vi "FTW-Regex.vi"(0 "Regular Expression":string, 5 "Input String":string, 9 "Starting Offset":i32, 11 "error in":errorcluster) -> (4 "Match":string, 6 "Submatches":string[](array[string]), 8 "Match Found?":bool, 10 "Offset after Match":i32, 15 "error out":errorcluster)   [LabVIEW 2015]
uses:
  error/FTW-ERR-ThrowGenericError.vi
  error/FTW-ERR-ThrowError.vi
  error/FTW-ERR-CallChain.vi
  error/FTW-ERR-NoErrorConstant.vi
  string/FTW-STR-ReplaceWhitespace.vi
  string/FTW-STR-Array-Delimit.vi
  error/FTW-ERR-Clear.vi
  FTW-Regex-ReplaceAll.vi
  lib/FTW-KernelFilepath.vi
panel:
  # "Inputs"
  # "Debug"
  # "Outputs"
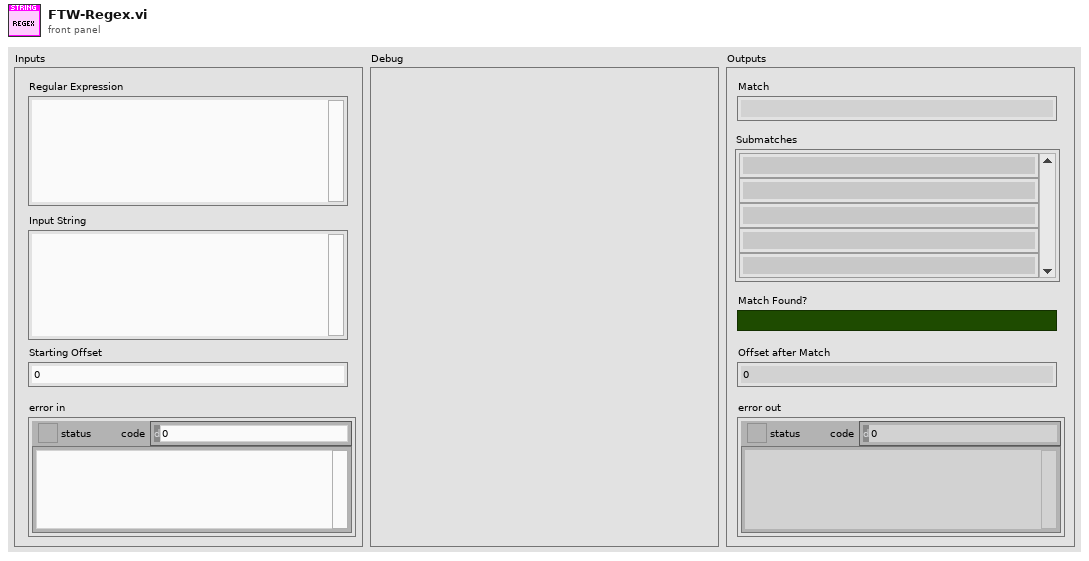
[diagram p1: front panel]
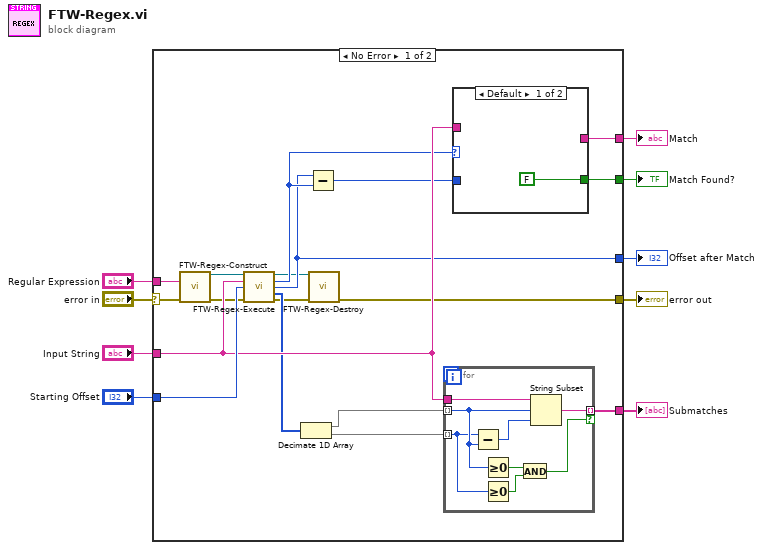
[diagram p0: block diagram]
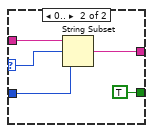
[diagram p2: hidden frame]
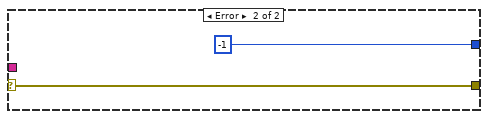
[diagram p3: hidden frame]
diagram:
  n1 = case shown="No Error" "error in" {
    selector: "error in" -> [w20 w42]
    tunnel: "Regular Expression" -> [w27 _]
    tunnel: [w26 _] -> w8
    tunnel: [w25 _] -> w7
    tunnel: [w10 w42] -> w6
    tunnel: "Starting Offset" -> [w24 _]
    tunnel: [w18 -1] -> w4
    tunnel: [w23 _] -> w3
    tunnel: "Input String" -> [w22 _]
    frame No Error {
      n2 = call "FTW-Regex-Construct.vi"("Regular Expression"=w27, "error in"=w20) -> ("Regex"=w14:refnum<data-value>, "error out"=w16:errorcluster)  [unwired: 12 in]
      n3 = call "FTW-Regex-Execute.vi"("Regex"=w14, "Subject String"=w22, "Starting Offset"=w24, "error in"=w16) -> ("Regex out"=w15:refnum<data-value>, "Whole Match Begin"=w19:i32, "Offset after Match"=w18:i32, "Submatches"=w21:i32[], "error out"=w17:errorcluster)  [unwired: 6 in, 1 out]
      n4 = Decimate 1D Array(w21) -> (w13:i32[], w12:i32[])
      n5 = Subtract(x=w18, y=w19) -> (x-y=w11:i32)
      n6 = call "FTW-Regex-Destroy.vi"("Regex"=w15, "error in"=w17) -> ("error out"=w10:errorcluster)  [unwired: 13 in]
      n7 = for {
        tunnel: w22 -> [w41]
        tunnel: [w40] -> w25 mode=indexing if=w35
        tunnel: w13 -> [w38] mode=indexing
        tunnel: w12 -> [w34] mode=indexing
        n8 = Subtract(x=w34, y=w38) -> (x-y=w39:i32)
        n9 = Greater Or Equal To 0?(x=w38) -> (x >= 0?=w37:bool)
        n10 = Greater Or Equal To 0?(x=w34) -> (x >= 0?=w36:bool)
        n11 = And(x=w37, y=w36) -> (x .and. y?=w35:bool)
        n12 = String Subset(string=w41, offset (0)=w38, length (rest)=w39) -> (substring=w40:string)
      }
      n13 = case shown="Default" w19 {
        selector: w19 -> [_ w30]
        tunnel: w22 -> [_ w33]
        tunnel: [_ w32] -> w26
        tunnel: w11 -> [_ w31]
        tunnel: [FALSE TRUE] -> w23
        frame Default {
        }
        frame 0.. {
          n14 = String Subset(string=w33, offset (0)=w30, length (rest)=w31) -> (substring=w32:string)
        }
      }
    }
    frame Error {
    }
  }
  "error out" <- w6
  "Submatches" <- w7
  "Match" <- w8
  "Match Found?" <- w3
  "Offset after Match" <- w4
